vi "Actor Core.vi"(8 "error in":errorcluster, 11 "Keepalive Heartbeat in":refnum<class "Keepalive Heartbeat.lvclass">) -> (0 "error out":errorcluster, 3 "Actor out":refnum<class "Actor.lvclass">)   [LabVIEW 2021, in "WebSocket Actors.lvlib" / "Keepalive Heartbeat.lvclass"]
doc: "(<B>Filename</B>: Actor Framework.lvlib:Actor.lvclass:Actor Core.vi)\n\nReceives messages to the actor, reacts to them, and initiates any error handling that may shut the actor down.\n\nDescendant classes may override this VI to append parallel tasks for the actor to complete while it handles messages. Overrides use the Call Parent Class Method node."
uses:
  Keepalive Heartbeat.lvclass
  C:/Program Files/National Instruments/LabVIEW 2021/vi.lib/ActorFramework/Actor/Actor.lvclass
  <vilib>/ActorFramework/Actor/Actor.lvclass
  <vilib>/ActorFramework/Actor/Actor.lvclass/Actor.ctl
  <vilib>/ActorFramework/Message Enqueuer/Message Enqueuer.lvclass/Message Enqueuer.ctl
  Keepalive Heartbeat.lvclass/Keepalive Heartbeat.ctl
  <vilib>/ActorFramework/Message Enqueuer/Init from Existing Queue.vi
  <vilib>/ActorFramework/Message Enqueuer/Enqueue.vi
  <vilib>/ActorFramework/Stop Msg/Stop Msg.lvclass
  C:/Program Files/National Instruments/LabVIEW 2021/vi.lib/ActorFramework/Message/Message.lvclass
  <vilib>/Utility/LVClass/Get LV Class Name.vi
  <resource>/AFDebug/Generate Trace for Message.vi
  <vilib>/ActorFramework/Message Priority Queue/Priority Enqueue.vi
  <vilib>/ActorFramework/Message Enqueuer/Message Enqueuer.lvclass
  WebSocket Connection Messages/Send Ping Msg/Send Ping Msg.lvclass
  C:/Projects/WebSocket-Actor/WebSocket Actor/Keepalive Heartbeat/Keepalive Heartbeat.lvclass
  WebSocket Connection Messages/Drop Connection Msg/Drop Connection Msg.lvclass
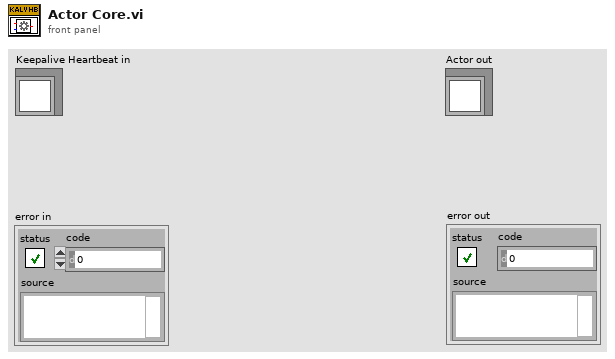
[diagram p1: front panel]
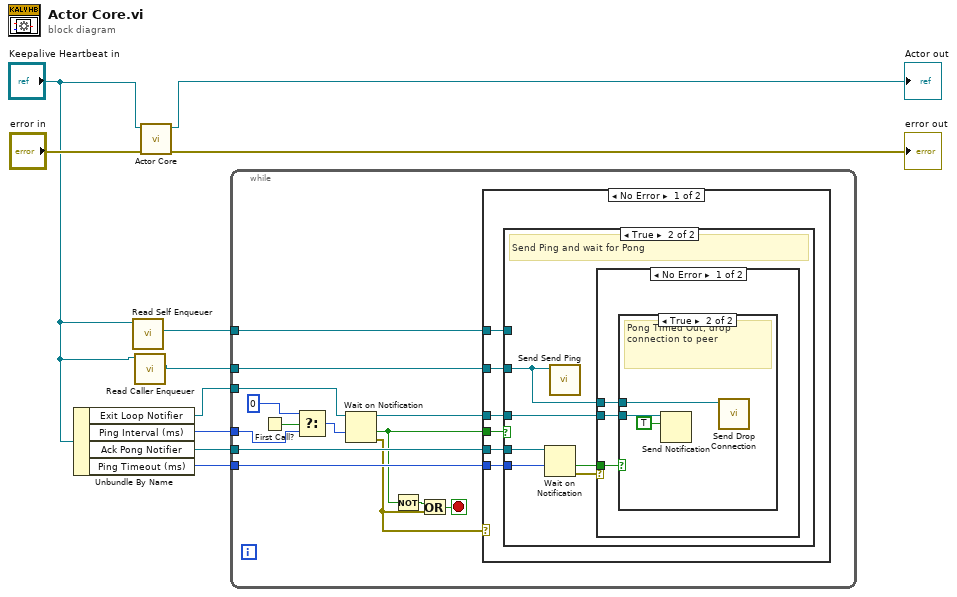
[diagram p0: block diagram]
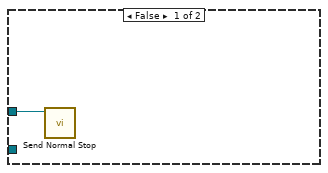
[diagram p2: hidden frame]
diagram:
  n1 = Unbundle By Name("Keepalive Heartbeat in") -> ("Exit Loop Notifier"=w7:refnum<notifier>, "Ping Interval (ms)"=w6:u32, "Ack Pong Notifier"=w1:refnum<notifier>, "Ping Timeout (ms)"=w2:u32)
  n2 = call <vilib>:"Read Self Enqueuer.vi"("Actor"="Keepalive Heartbeat in") -> ("Self Enqueuer"=w3:refnum<class "Message Enqueuer.lvclass">)  [unwired: 10 in]
  n3 = call <vilib>:"Read Caller Enqueuer.vi"("Actor"="Keepalive Heartbeat in") -> ("Caller Enqueuer"=w5:refnum<class "Message Enqueuer.lvclass">)  [unwired: 10 in]
  n4 = call-parent "Actor Core.vi"("error in"="error in", "Actor in"="Keepalive Heartbeat in") -> ("error out"=→"error out":errorcluster, "Actor out"=→"Actor out":refnum<class "Actor.lvclass">)  [unwired: 8 in]
  n5 = while {
    tunnel: w7 -> [w24]
    tunnel: w6 -> [w13]
    tunnel: w5 -> [w23]
    tunnel: w3 -> [w22]
    tunnel: w2 -> [w21]
    tunnel: w1 -> [w20]
    stop <- w17 stop-if-true
    n6 = First Call?() -> (First Call?: T/F=w14:bool)
    n7 = Select(t=u32 0, s=w14, f=w13) -> (s? t:f=w11:u32)
    n8 = Wait on Notification(notifier=w24, timeout in ms (-1)=w11) -> (notifier out=w19:refnum<notifier>, timed out?=w18:bool, error out=w16:errorcluster)  [unwired: 2 in, 1 out]
    n9 = Not(x=w18) -> (.not. x?=w15:bool)
    n10 = Or(x=w15, y=w16) -> (x .or. y?=w17:bool)
    n11 = case shown="No Error" w16 {
      tunnel: w23 -> [w30 _]
      tunnel: w18 -> [w29 _]
      tunnel: w22 -> [w28 _]
      tunnel: w21 -> [w27 _]
      tunnel: w20 -> [w26 _]
      tunnel: w19 -> [w25 _]
      frame No Error {
        n12 = case shown="True" w29 {
          tunnel: w30 -> [_ w33]
          tunnel: w28 -> [w31 _]
          tunnel: w27 -> [_ w37]
          tunnel: w26 -> [_ w36]
          tunnel: w25 -> [_ w34]
          frame False {
            n13 = call <vilib>:"Send Normal Stop.vi"("Message Enqueuer"=w31) -> ()  [unwired: 10 in, 1 out]
          }
          frame True {
            # "Send Ping and wait for Pong"
            n14 = Wait on Notification(notifier=w36, timeout in ms (-1)=w37) -> (timed out?=w35:bool, error out=w32:errorcluster)  [unwired: 2 in, 2 out]
            n15 = call "Send Send Ping.vi"("Message Enqueuer in"=w33) -> ()  [unwired: 9 in, 2 out]
            n16 = case shown="No Error" w32 {
              tunnel: w35 -> [w40 _]
              tunnel: w34 -> [w39 _]
              tunnel: w33 -> [w38 _]
              frame No Error {
                n17 = case shown="True" w40 {
                  tunnel: w39 -> [_ w43]
                  tunnel: w38 -> [_ w41]
                  frame False {
                  }
                  frame True {
                    # "Pong Timed Out, drop connection to peer"
                    n18 = Send Notification(notification=TRUE, notifier=w43) -> ()  [unwired: 1 in, 2 out]
                    n19 = call "Send Drop Connection.vi"("Message Enqueuer in"=w41) -> ()  [unwired: 9 in, 2 out]
                  }
                }
              }
              frame Error {
                # "The Actor Stop was called while waiting for the Pong"
              }
            }
          }
        }
      }
      frame Error {
        # "The Actor Stop was called and destroyed the exit notifier"
      }
    }
  }
